vi "NAQ_DO_COM.vi"() -> ()   [LabVIEW 2016, in "NAQ_DO.lvlib"]
uses:
  NAQ_DO.lvlib
panel:
  in  "停止":bool
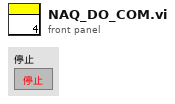
[diagram p1: front panel]
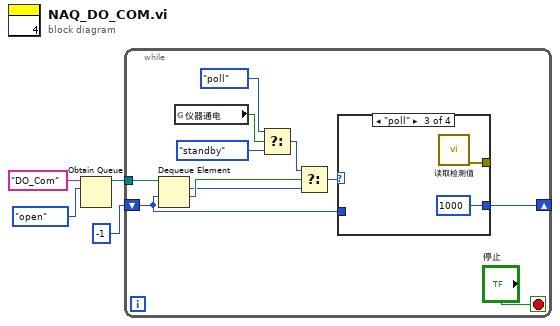
[diagram p0: block diagram]
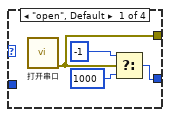
[diagram p2: hidden frame]
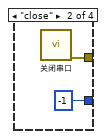
[diagram p3: hidden frame]
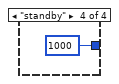
[diagram p4: hidden frame]
diagram:
  n1 = Obtain Queue(name (unnamed)="DO_Com" ("名称（未命名）"), element data type=enum16{"open", "close", "poll", "standby"}."open" ("枚举")) -> (queue out=w2:refnum<queue>)  [unwired: 3 in, 2 out]
  n2 = while {
    tunnel: w2 -> [w15]
    shift-right: [w6] -> _
    shift-left: -1 ("超时毫秒(-1)") -> [w5]
    stop <- "停止" stop-if-true
    n3 = Dequeue Element(queue=w15, timeout in ms (-1)=w5) -> (element=w9:enum16{"open", "close", "poll", "standby"}, timed out?=w13:bool)  [unwired: 1 in, 2 out]
    n4 = global read "过程变量.vi" "仪器通电"() -> (w12:bool)
    n5 = Select(t=enum16{"open", "close", "poll", "standby"}."poll" ("枚举"), s=w12, f=enum16{"open", "close", "poll", "standby"}."standby" ("枚举")) -> (s? t:f=w7:enum16{"open", "close", "poll", "standby"})
    n6 = Select(t=w7, s=w13, f=w9) -> (s? t:f=w10:enum16{"open", "close", "poll", "standby"})
    n7 = case shown="\"poll\"" w10 {
      tunnel: [w19 w21 w23 _] -> _
      tunnel: w5 -> [_ _ _ _]
      tunnel: [w16 -1 ("f") 1000 ("f") 1000 ("f")] -> w6
      frame "open", Default {
        n8 = call "打开串口.vi"() -> ("Error out"=w19:errorcluster)  [unwired: 11 in]
        n9 = Select(t=-1 ("超时毫秒(-1)"), s=w19, f=1000) -> (s? t:f=w16:i32)
      }
      frame "close" {
        n10 = call "关闭串口.vi"() -> ("error out"=w21:errorcluster)  [unwired: 11 in]
      }
      frame "poll" {
        n11 = call "读取检测值.vi"() -> ("error out"=w23:errorcluster)  [unwired: 10 in, 1 out]
      }
      frame "standby" {
      }
    }
  }
